vi "Enable Eager Loading.vi"   [LabVIEW 2020]
uses:
  User Interface/Execution UI/User Interface.vi
  User Interface/Execution UI/Execution UI.lvclass
panel:
  # "Eager Loading\nEager Loading has now been enabled by adding the LUnit Framework.lvlib to the project. You may remove it from your project at any time and the dependencies will then be loaded implicitly when needed.\n\nHow it works\nThe LUnit Execution UI is located in vi.lib and as default only loaded into memory when the launcher is called from the menu. By explicitly including the LUnit Framework.lvlib from vi.lib in the LabVIEW project, the needed files will be loaded into memory when the project is opened. This significantly reduces the loading time of the Execution UI and it is therefore recommended to keep this library in the project while developing in a workflow with frequent executions of unit tests.\n\nGood to know\nA drawback of explicitly including the LUnit Support.lvlib is that all classes used by the LUnit framework will be loaded into memory and will thus clutter the class hierarchy graph and the Create New Class dialog. There is also a slight increase in the load time of the LabVIEW project.\n\nClick anywhere to close this dialog."
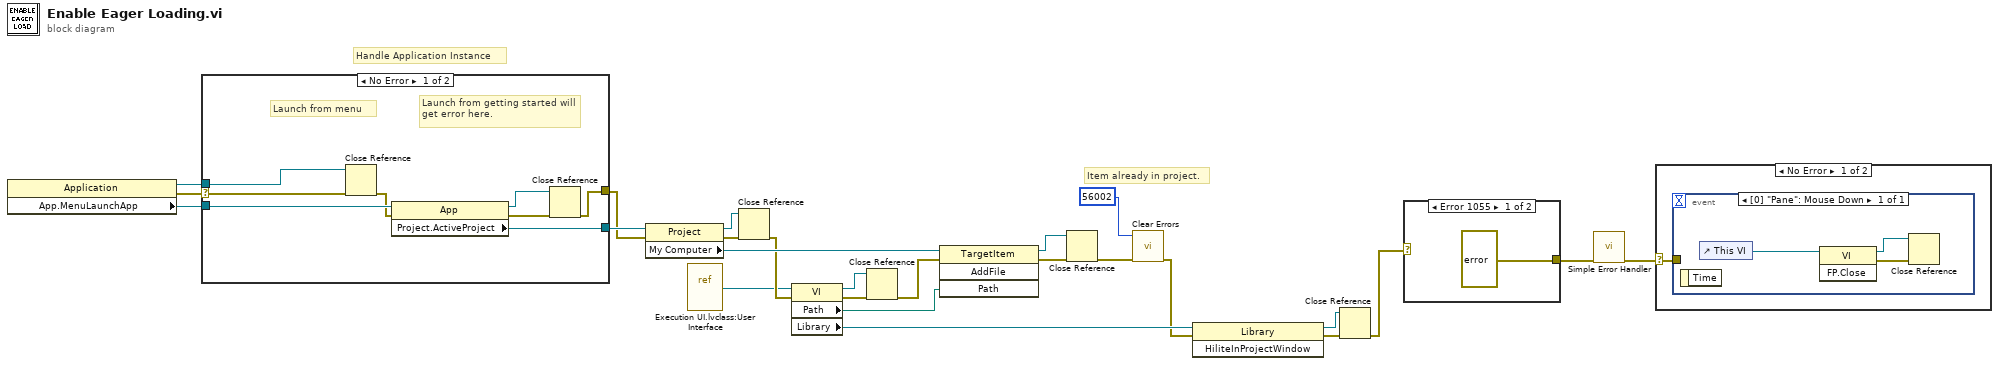
[diagram p0: block diagram]
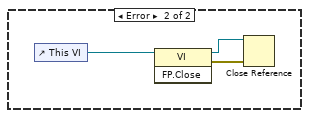
[diagram p2: hidden frame]
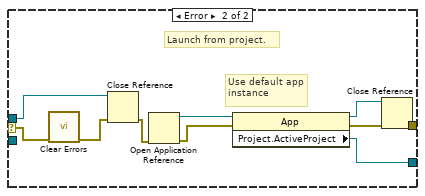
[diagram p3: hidden frame]
diagram:
  # "Item already in project."
  # "Handle Application Instance"
  n1 = property class="Application"() -> (reference out=w23:refnum<vi>, error out=w24:errorcluster, "App.MenuLaunchApp"=w25:refnum<vi>)  [unwired: 2 in]
  n2 = case shown="No Error" w24 {
    selector: w24 -> [w32 w41]
    tunnel: w25 -> [w31 _]
    tunnel: w23 -> [w33 w40]
    tunnel: [w27 w37] -> w22
    tunnel: [w26 w35] -> w21
    frame No Error {
      # "Launch from getting started will get error here."
      # "Launch from menu"
      n3 = Close Reference(reference=w33, error in (no error)=w32) -> (error out=w30:errorcluster)
      n4 = property class="App"(reference=w31, error in=w30) -> (reference out=w29:refnum<vi>, error out=w28:errorcluster, "Project.ActiveProject"=w27:refnum<vi>)
      n5 = Close Reference(reference=w29, error in (no error)=w28) -> (error out=w26:errorcluster)
    }
    frame Error {
      # "Launch from project."
      # "Use default app instance"
      n6 = call <vilib>:"Clear Errors.vi"("error in (no error)"=w41) -> ("error out"=w39:errorcluster)  [unwired: 5 in, 1 out]
      n7 = Close Reference(reference=w40, error in (no error)=w39) -> (error out=w38:errorcluster)
      n8 = Open Application Reference(8:w38) -> (0:w42:errorcluster, 3:w43:refnum<vi>)  [unwired: 3 in]
      n9 = property class="App"(reference=w43, error in=w42) -> (reference out=w34:refnum<vi>, error out=w36:errorcluster, "Project.ActiveProject"=w37:refnum<vi>)
      n10 = Close Reference(reference=w34, error in (no error)=w36) -> (error out=w35:errorcluster)
    }
  }
  n11 = property class="Project"(reference=w22, error in=w21) -> (reference out=w19:refnum<vi>, error out=w18:errorcluster, "My Computer"=w20:refnum<vi>)
  n12 = vi-ref "Execution UI.lvclass:User Interface.vi"() -> (w4:refnum<vi>)
  n13 = Close Reference(reference=w19, error in (no error)=w18) -> (error out=w12:errorcluster)
  n14 = property class="VI"(reference=w4, error in=w12) -> (reference out=w13:refnum<vi>, error out=w14:errorcluster, "Path"=w15:path, "Library"=w8:refnum<vi>)
  n15 = Close Reference(reference=w13, error in (no error)=w14) -> (error out=w11:errorcluster)
  n16 = invoke class="TargetItem" method="AddFile"(reference=w20, error in=w11, "Path"=w15) -> (reference out=w16:refnum<vi>, error out=w17:errorcluster)  [unwired: 1 in, 2 out]
  n17 = Close Reference(reference=w16, error in (no error)=w17) -> (error out=w10:errorcluster)
  n18 = call <vilib>:"Clear Errors.vi"("error in (no error)"=w10, "specific error code to clear (0: all)"=56002) -> ("error out"=w5:errorcluster)  [unwired: 4 in, 1 out]
  n19 = invoke class="Library" method="HiliteInProjectWindow"(reference=w8, error in=w5) -> (reference out=w6:refnum<vi>, error out=w7:errorcluster)  [unwired: 1 in, 1 out]
  n20 = Close Reference(reference=w6, error in (no error)=w7) -> (error out=w2:errorcluster)
  n21 = case shown="Error 1055" w2 {
    selector: w2 -> [_ w45]
    tunnel: [errorcluster {"status"=TRUE, "code"=1546, "source"="Eager loading can only be activated from within a LabVIEW Project. Please create a project file before activating eager loading."} ("error out") w45] -> w1
    frame #0 {
    }
    frame #1 {
    }
  }
  n22 = call <vilib>:"Simple Error Handler.vi"("error in (no error)"=w1) -> ("error out"=w3:errorcluster)  [unwired: 4 in, 4 out]
  n23 = case shown="No Error" w3 {
    selector: w3 -> [w46 _]
    frame No Error {
      n24 = event shown="[0] \"Pane\": Mouse Down" {
        selector: _ -> [_]
        dyn-events: _ -> [_]
        timeout: _ -> [_]
        tunnel: w46 -> [_]
        event Mouse Down {
          n25 = event-data() -> ()  [unwired: 1 in, 1 out]
          n26 = control-ref of="This VI"() -> (w47:refnum<vi>)
          n27 = invoke class="VI" method="FP.Close"(reference=w47) -> (reference out=w49:refnum<vi>, error out=w48:errorcluster)  [unwired: 2 in, 1 out]
          n28 = Close Reference(reference=w49, error in (no error)=w48) -> ()  [unwired: 1 out]
        }
      }
    }
    frame Error {
      n29 = control-ref of="This VI"() -> (w50:refnum<vi>)
      n30 = invoke class="VI" method="FP.Close"(reference=w50) -> (reference out=w52:refnum<vi>, error out=w51:errorcluster)  [unwired: 2 in, 1 out]
      n31 = Close Reference(reference=w52, error in (no error)=w51) -> ()  [unwired: 1 out]
    }
  }
